vi "適應性控制_線上學習_V6(實際控制).vi"() -> ()   [LabVIEW 2010]
uses:
  <vilib>/DAQmx/read.llb/DAQmx Read (Analog 1D Wfm NChan NSamp).vi
  <vilib>/DAQmx/write.llb/DAQmx Write (Analog DBL 1Chan 1Samp).vi
  <vilib>/DAQmx/create/channels.llb/DAQmx Create Channel (AI-Voltage-Basic).vi
  <vilib>/DAQmx/configure/timing.llb/DAQmx Timing (Sample Clock).vi
  <vilib>/DAQmx/create/channels.llb/DAQmx Create Channel (AO-Voltage-Basic).vi
  <vilib>/daqmx/miscellaneous.llb/DAQmx Fill In Error Info.vi
panel:
  in  "電路 channels":tag="PXI-6229/ai1"
  in  "加速規 channels":tag="PXI-6229/ai0"
  out "輸入訊號":dbl[][](graph)
  out "輸出是否超過範圍":bool
  out "while平均執行時間(ms)":dbl
  out "Time (s)":dbl caption="Elapsed Time (s)"
  out "Waveform Chart 2":dbl(graph)
  in  "error in":errorcluster
  in  "DAQ output":tag="PXI-6733/ao3"
  out "source out":string
  out "當下誤差":dbl=0.1 format="%#_13g"
  out "理想與FIR輸出":dbl[][](graph)
  out "誤差":dbl(graph)
  out "權重(w)":dbl[](array[numeric])
  in  "收斂係數":dbl=0.0001
  in  "order":i32=150
  in  "\"每\"通道取樣頻率":dbl=1000.0 min=1.0 max=10000.0 step=1.0
  in  "stop":bool
  # "多通道採樣時,原本輸入的取樣頻率會隨通道數多寡被平均掉"
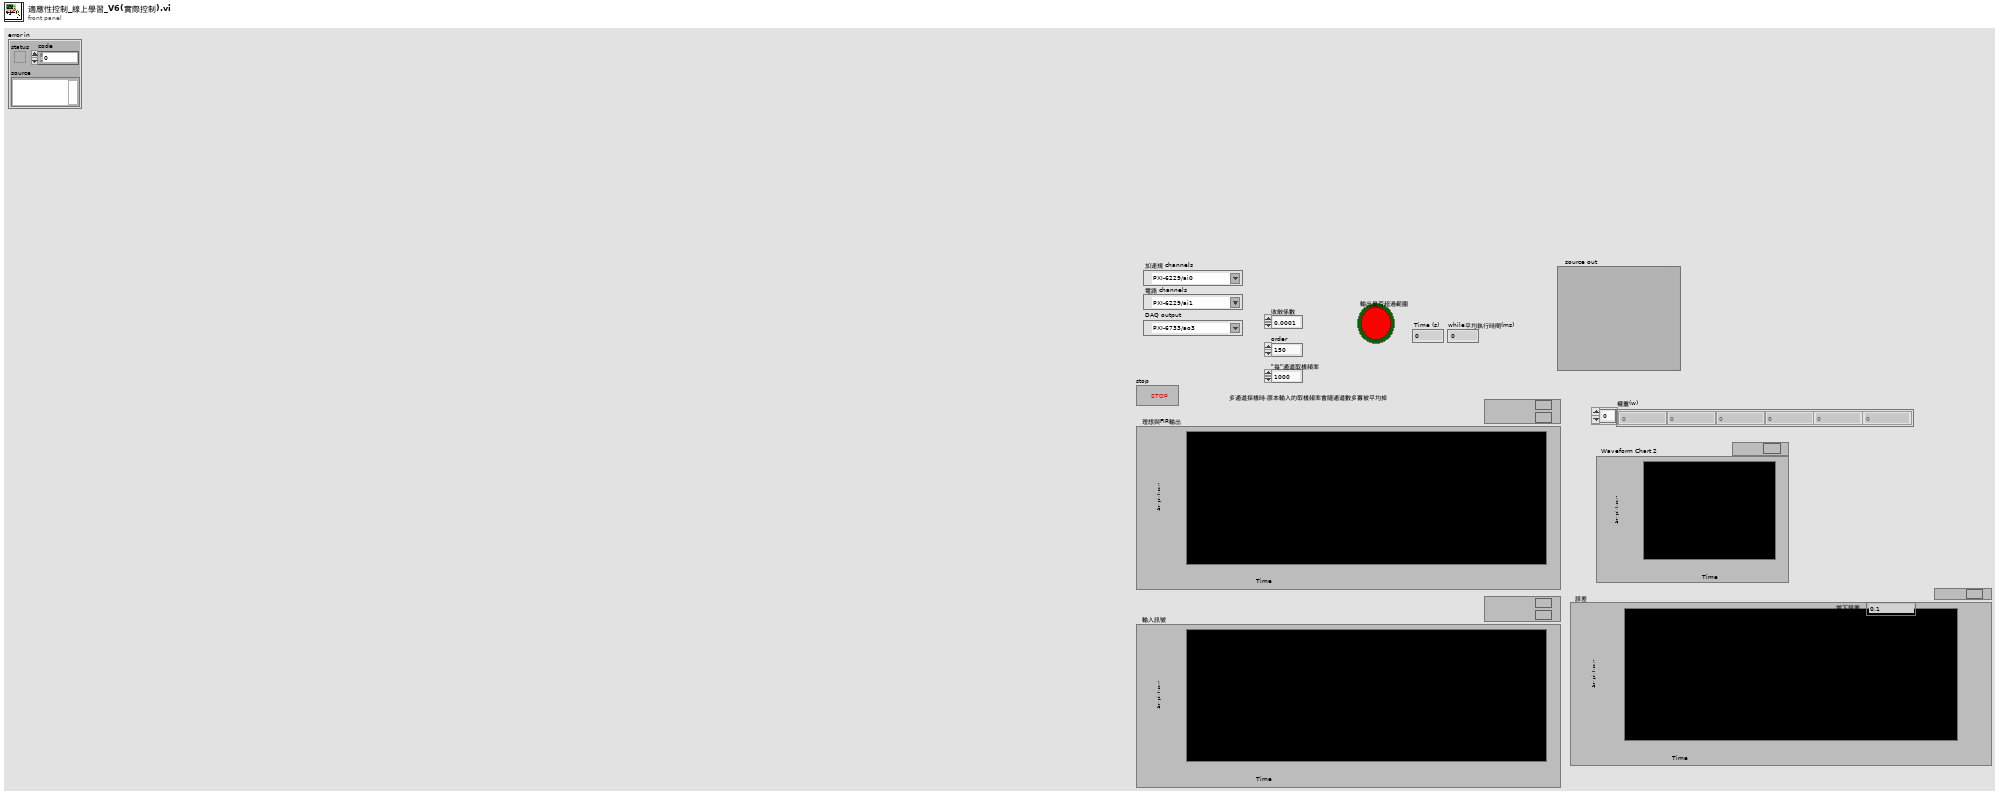
[diagram p1: front panel]
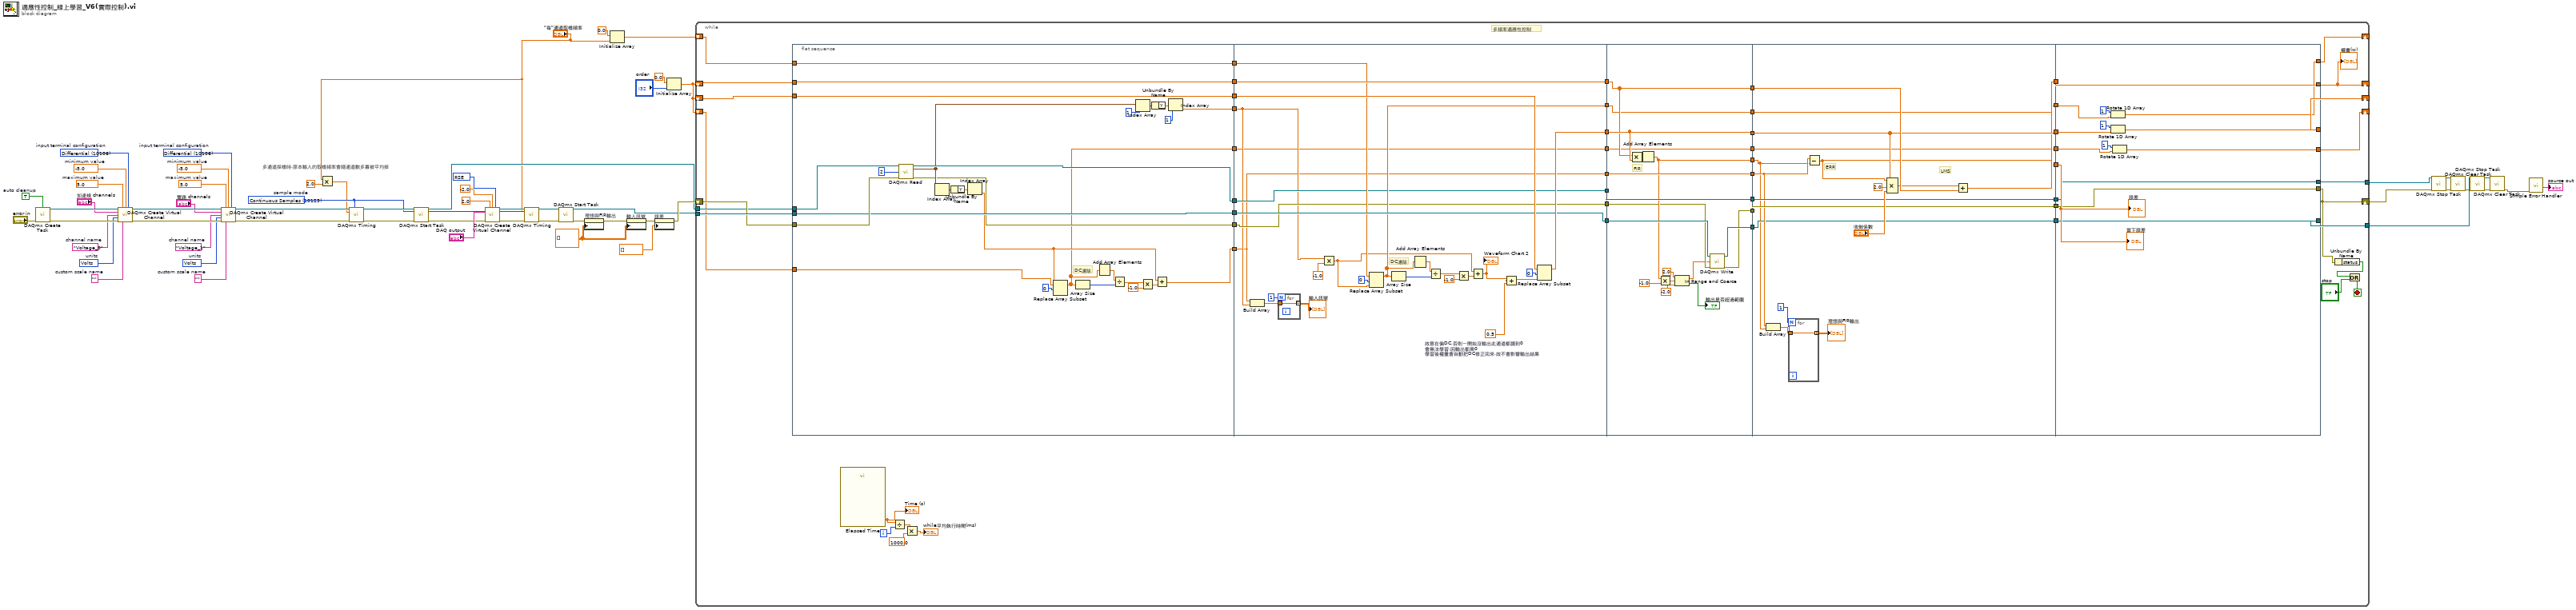
[diagram p0: block diagram]
diagram:
  w16 = 10123 items=["Finite Samples"=10178, "Continuous Samples"=10123, "Hardware Timed Single Point"=12522]  # sample mode
  w19 = 10106 items=["default"=-1, "RSE"=10083, "NRSE"=10078, "Differential"=10106, "Pseudodifferential"=12529]  # input terminal configuration
  w20 = 10348 items=["Volts"=10348, "From Custom Scale"=10065]  # units
  w21 = "Voltage_1"  # channel name
  w23 = ""  # custom scale name
  w24 = -5.0  # minimum value
  w25 = 5.0  # maximum value
  w26 = 10106 items=["default"=-1, "RSE"=10083, "NRSE"=10078, "Differential"=10106, "Pseudodifferential"=12529]  # input terminal configuration
  w27 = 10348 items=["Volts"=10348, "From Custom Scale"=10065]  # units
  w28 = "Voltage_0"  # channel name
  w30 = ""  # custom scale name
  w31 = -5.0  # minimum value
  w32 = 5.0  # maximum value
  w34 = TRUE  # auto cleanup
  w53 = 10083 items=["Default"=-1, "RSE"=10083, "Differential"=10106, "Pseudodifferential"=12529] ("output terminal configuration")
  w4 = dbl[][] [] ("History Data")
  # "多通道採樣時,原本輸入的取樣頻率會隨通道數多寡被平均掉"
  n1 = call <vilib>:"DAQmx Create Task.vi"("auto cleanup"=w34, "error in"="error in") -> ("task out"=w33:refnum<k21>, "error out"=w35:errorcluster)  [unwired: 12 in]
  n2 = call-poly <vilib>:"DAQmx Create Virtual Channel.vi"("task in"=w33, "maximum value"=w32, "minimum value"=w31, "input terminal configuration"=w26, "physical channels"="加速規 channels", "name to assign"=w28, "units"=w27, "error in"=w35, "custom scale name"=w30) -> ("task out"=w12:refnum<k21>, "error out"=w29:errorcluster)  [unwired: 5 in]
  n3 = call-poly <vilib>:"DAQmx Create Virtual Channel.vi"("task in"=w12, "maximum value"=w25, "minimum value"=w24, "input terminal configuration"=w19, "physical channels"="電路 channels", "name to assign"=w21, "units"=w20, "error in"=w29, "custom scale name"=w23) -> ("task out"=w18:refnum<k21>, "error out"=w22:errorcluster)  [unwired: 5 in]
  n4 = Multiply(x="\"每\"通道取樣頻率", y=2.0) -> (x*y=w1:dbl)
  n5 = call-poly <vilib>:"DAQmx Timing.vi"("task/channels in"=w18, "sample mode"=w16, "rate"=w1, "error in"=w22) -> ("task out"=w17:refnum<k21>, "error out"=w13:errorcluster)  [unwired: 10 in]
  n6 = call <vilib>:"DAQmx Start Task.vi"("task/channels in"=w17, "error in"=w13) -> ("task out"=w14:refnum<k21>, "error out"=w40:errorcluster)  [unwired: 12 in]
  n7 = call-poly <vilib>:"DAQmx Create Virtual Channel.vi"("maximum value"=2.0, "minimum value"=-2.0, "output terminal configuration"=w53, "physical channels"="DAQ output", "error in"=w40) -> ("task out"=w54:refnum<k21>, "error out"=w57:errorcluster)  [unwired: 9 in]
  n8 = call-poly <vilib>:"DAQmx Timing.vi"("task/channels in"=w54, "sample mode"=w16, "rate"="\"每\"通道取樣頻率", "error in"=w57) -> ("task out"=w55:refnum<k21>, "error out"=w56:errorcluster)  [unwired: 10 in]
  n9 = call <vilib>:"DAQmx Start Task.vi"("task/channels in"=w55, "error in"=w56) -> ("task out"=w10:refnum<k21>, "error out"=w15:errorcluster)  [unwired: 12 in]
  n10 = property on="理想與FIR輸出" class="WFChart (strict)"(error in=w15, "History Data"=w4) -> (error out=w6:errorcluster)  [unwired: 1 in, 1 out]
  n11 = Initialize Array(0.0 ("element"), "\"每\"通道取樣頻率") -> (w41:dbl[])
  n12 = property on="輸入訊號" class="WFChart (strict)"(error in=w6, "History Data"=w4) -> (error out=w5:errorcluster)  [unwired: 1 in, 1 out]
  n13 = property on="誤差" class="WFChart (strict)"(error in=w5, "History Data"=dbl[] []) -> (error out=w38:errorcluster)  [unwired: 1 in, 1 out]
  n14 = Initialize Array(0.0 ("element"), "order") -> (w9:dbl[])
  n15 = while {
    shift-right: [w103] -> _
    shift-left: w9 -> [w115]
    shift-right: [w107] -> _
    shift-left: w9 -> [w111]
    tunnel: w10 -> [w102]
    tunnel: [w88] -> w48
    tunnel: [w87] -> w47
    shift-right: [w74] -> _
    shift-left: w41 -> [w84]
    tunnel: w14 -> [w76]
    shift-right: [w75] -> w11
    shift-left: w38 -> [w101]
    shift-right: [w65] -> _
    shift-left: w9 -> [w66]
    i -> [w70]
    stop <- w85 stop-if-true
    # "多頻率適應性控制"
    n16 = flat-sequence {
      tunnel: [w143] -> w116
      tunnel: w115 -> [w143]
      tunnel: [w142] -> w112
      tunnel: w111 -> [w142]
      tunnel: w102 -> [w128]
      tunnel: w101 -> [w140]
      tunnel: [w139] -> w100
      tunnel: [w127] -> w99
      tunnel: [w128] -> w92
      tunnel: w84 -> [w141]
      tunnel: [w141] -> w83
      tunnel: w76 -> [w130]
      tunnel: [w131] -> w73
      tunnel: [w118] -> w72
      tunnel: w66 -> [w120]
      tunnel: [w117] -> w61
      tunnel: w116 -> [w167]
      tunnel: [w169] -> w114
      tunnel: [w168] -> w113
      tunnel: w112 -> [w168]
      tunnel: w100 -> [w155]
      tunnel: w99 -> [w154]
      tunnel: [w154] -> w98
      tunnel: [w155] -> w95
      tunnel: [w165] -> w93
      tunnel: w92 -> [w165]
      tunnel: w83 -> [w159]
      tunnel: [w158] -> w82
      tunnel: [w149] -> w77
      tunnel: w73 -> [w152]
      tunnel: w72 -> [w149]
      tunnel: [w148] -> w62
      tunnel: w61 -> [w148]
      tunnel: w114 -> [w186]
      tunnel: w113 -> [w185]
      tunnel: [w185] -> w110
      tunnel: [w174] -> w109
      tunnel: [w186] -> w108
      tunnel: w98 -> [w173]
      tunnel: [w172] -> w97
      tunnel: w95 -> [w187]
      tunnel: [w187] -> w94
      tunnel: w93 -> [w178]
      tunnel: [w177] -> w91
      tunnel: w82 -> [w184]
      tunnel: [w184] -> w81
      tunnel: [w183] -> w78
      tunnel: w77 -> [w183]
      tunnel: [w176] -> w63
      tunnel: w62 -> [w176]
      tunnel: w110 -> [w205]
      tunnel: w109 -> [w189]
      tunnel: w108 -> [w201]
      tunnel: [w199] -> w106
      tunnel: [w201] -> w105
      tunnel: [w193] -> w104
      tunnel: w97 -> [w198]
      tunnel: [w198] -> w96
      tunnel: w94 -> [w197]
      tunnel: w91 -> [w192]
      tunnel: [w192] -> w90
      tunnel: [w197] -> w89
      tunnel: w81 -> [w196]
      tunnel: [w196] -> w80
      tunnel: w78 -> [w194]
      tunnel: [w190] -> w64
      tunnel: w63 -> [w190]
      tunnel: [w220] -> w107
      tunnel: w106 -> [w220]
      tunnel: w105 -> [w217]
      tunnel: [w219] -> w103
      tunnel: w104 -> [w216]
      tunnel: w96 -> [w215]
      tunnel: [w215] -> w75
      tunnel: w90 -> [w213]
      tunnel: w89 -> [w214]
      tunnel: [w214] -> w88
      tunnel: [w213] -> w87
      tunnel: [w210] -> w74
      tunnel: w80 -> [w211]
      tunnel: [w208] -> w65
      tunnel: w64 -> [w207]
      frame #0 {
        # "DC濾除"
        n17 = call-poly <vilib>:"DAQmx Read.vi"("task/channels in"=w130, "number of samples per channel"=2, "error in"=w140) -> ("task out"=w139:refnum<k21>, "data"=w132:waveform(dbl)[], "error out"=w127:errorcluster)  [unwired: 10 in]
        n18 = Index Array(array=w132) -> (element=w138:waveform(dbl))  [unwired: 1 in]
        n19 = Unbundle By Name(w138) -> ("Y"=w137:dbl[])
        n20 = Index Array(array=w137) -> (element=w119:dbl)  [unwired: 1 in]
        n21 = Replace Array Subset(array=w120, new element=w119, index=0) -> (w117:dbl[])
        n22 = Array Size(array=w117) -> (size(s)=w124:i32)
        n23 = Add Array Elements(numeric array=w117) -> (sum=w123:dbl)
        n24 = Divide(x=w123, y=w124) -> (x/y=w125:dbl)
        n25 = Index Array(array=w132, index=1) -> (element=w136:waveform(dbl))
        n26 = Multiply(x=w125, y=-1.0) -> (x*y=w126:dbl)
        n27 = Unbundle By Name(w136) -> ("Y"=w135:dbl[])
        n28 = Add(x=w119, y=w126) -> (x+y=w118:dbl)
        n29 = Index Array(array=w135, index=1) -> (element=w131:dbl)
      }
      frame #1 {
        w146 = 0.5  # 故意在偏DC,否則一開始沒輸出此通道都讀到0 會無法學習,因輸出都乘0 學習後權重會自動把DC修正回來,故不會影響輸出結果
        # "DC濾除"
        n30 = Build Array(w149, w152) -> (w151:dbl[])
        n31 = for {
          N: 1 -> [_]
          tunnel: w151 -> [w170]
          tunnel: [w170] -> w144 mode=indexing
        }
        "輸入訊號" <- w144
        n32 = Multiply(x=w152, y=-1.0) -> (x*y=w153:dbl)
        n33 = Replace Array Subset(array=w159, new element=w153, index=0) -> (w158:dbl[])
        n34 = Array Size(array=w158) -> (size(s)=w162:i32)
        n35 = Add Array Elements(numeric array=w158) -> (sum=w161:dbl)
        n36 = Divide(x=w161, y=w162) -> (x/y=w163:dbl)
        n37 = Multiply(x=w163, y=-1.0) -> (x*y=w164:dbl)
        n38 = Add(x=w153, y=w164) -> (x+y=w147:dbl)
        "Waveform Chart 2" <- w147
        n39 = Add(x=w147, y=w146) -> (x+y=w145:dbl)
        n40 = Replace Array Subset(array=w167, new element=w145, index=0) -> (w169:dbl[])
      }
      frame #2 {
        # "FIR"
        n41 = Multiply(x=w185, y=w186) -> (x*y=w188:dbl[])
        n42 = Add Array Elements(numeric array=w188) -> (sum=w174:dbl)
        n43 = Multiply(x=w174, y=-1.0) -> (x*y=w181:dbl)
        n44 = In Range and Coerce(upper limit=2.0, x=w181, lower limit=-2.0 ("upper limit")) -> (coerced(x)=w171:dbl, In Range?=→"輸出是否超過範圍":bool)
        n45 = call-poly <vilib>:"DAQmx Write.vi"("task/channels in"=w178, "data"=w171, "error in"=w173) -> ("task out"=w177:refnum<k21>, "error out"=w172:errorcluster)  [unwired: 10 in, 1 out]
      }
      frame #3 {
        # "LMS"
        # "ERR"
        n46 = Build Array(w194, w189) -> (w204:dbl[])
        n47 = for {
          N: 1 -> [_]
          tunnel: [w206] -> w191 mode=indexing
          tunnel: w204 -> [w206]
        }
        "理想與FIR輸出" <- w191
        n48 = Subtract(x=w194, y=w189) -> (x-y=w193:dbl)
        n49 = Compound Arithmetic op=MULTIPLY(w193, w201, 2.0, "收斂係數") -> (w200:dbl[])
        n50 = Add(x=w200, y=w205) -> (x+y=w199:dbl[])
      }
      frame #4 {
        n51 = Rotate 1D Array(1:w211, 2:1 ("n")) -> (0:w210:dbl[])
        n52 = Rotate 1D Array(1:w217, 2:1 ("n")) -> (0:w219:dbl[])
        n53 = Rotate 1D Array(1:w207, 2:1 ("n")) -> (0:w208:dbl[])
        "誤差" <- w216
        "當下誤差" <- w216
      }
    }
    n54 = call "Elapsed Time"() -> ("Elapsed Time (s)"=w71:dbl)  [unwired: 12 in, 7 out]
    "Time (s)" <- w71
    n55 = Divide(x=w71, y=w70) -> (x/y=w69:dbl)
    n56 = Multiply(x=w69, y=1000.0) -> (x*y=→"while平均執行時間(ms)":dbl)
    n57 = Unbundle By Name(w75) -> ("status"=w79:bool)
    n58 = Or(x=w79, y="stop") -> (x .or. y?=w85:bool)
    "權重(w)" <- w107
  }
  n59 = call <vilib>:"DAQmx Stop Task.vi"("task/channels in"=w48, "error in"=w11) -> ("task out"=w50:refnum<k21>, "error out"=w49:errorcluster)  [unwired: 12 in]
  n60 = call <vilib>:"DAQmx Clear Task.vi"("task in"=w50, "error in"=w49) -> ("error out"=w39:errorcluster)  [unwired: 13 in]
  n61 = call <vilib>:"DAQmx Stop Task.vi"("task/channels in"=w47, "error in"=w39) -> ("task out"=w45:refnum<k21>, "error out"=w46:errorcluster)  [unwired: 12 in]
  n62 = call <vilib>:"DAQmx Clear Task.vi"("task in"=w45, "error in"=w46) -> ("error out"=w37:errorcluster)  [unwired: 13 in]
  n63 = call <vilib>:"Simple Error Handler.vi"("error in (no error)"=w37) -> ("source out"=→"source out":string)  [unwired: 4 in, 4 out]
